vi "important information-autoConn.vi"() -> ()   [LabVIEW 2011]
panel:
  in  "ok":bool
  out "tip":string="    勾选后，USB掉线重启后，系统会自动以上一次配置启动设备。\n    主要应用于工业环境，提高可靠性，保证CAN调试器不间断运行。\n    系统不再弹出配置对话框，若要更改配置，请去掉勾选，重新启动设备。" caption="重要提示："
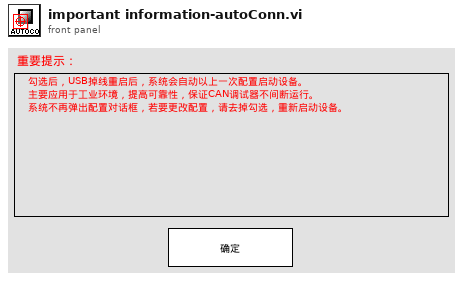
[diagram p1: front panel]
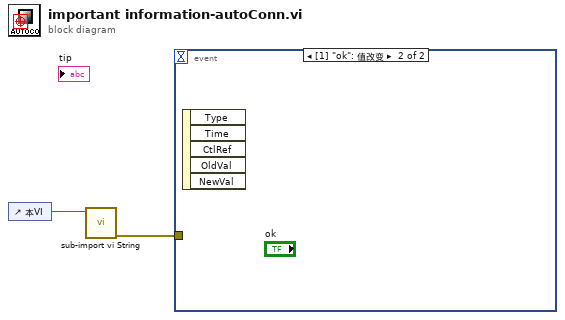
[diagram p0: block diagram]
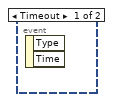
[diagram p2: hidden frame]
diagram:
  n1 = control-ref of="本VI"() -> (w2:refnum<vi>)
  n2 = call "sub-import vi String.vi"("vi ref"=w2) -> ("error out"=w1:errorcluster)  [unwired: 10 in]
  n3 = event shown="[1] \"ok\": 值改变" {
    selector: _ -> [_ _]
    dyn-events: _ -> [_ _]
    timeout: _ -> [_ _]
    tunnel: w1 -> [_ _]
    event Timeout {
      n4 = event-data() -> ()  [unwired: 1 in, 2 out]
    }
    event "ok": Value Change {
      n5 = event-data() -> ()  [unwired: 1 in, 5 out]
    }
  }
